vi "Initialize.vi"(8 "error in (no error)":errorcluster, 11 "Thread User Interface in":refnum<class "Thread User Interface.lvclass">) -> (0 "error out":errorcluster, 3 "Thread User Interface out":refnum<class "Thread User Interface.lvclass">)   [LabVIEW 2020, in "GE Reflective Memory.lvlib" / "Thread User Interface.lvclass"]
uses:
  Thread User Interface.lvclass
  Configurations/Thread/Thread Configuration.lvclass
  DSF Core.lvlibp/Classes/User Interface/User Interface.lvclass
  C:/Users/nitest/Desktop/Git 2020/niveristand-data-sharing-framework-custom-device-plugins/Components/DSF Core.lvlibp/Classes/Configuration/Configuration.lvclass
  C:/Users/nitest/Desktop/Git 2020/niveristand-data-sharing-framework-custom-device-plugins/Components/DSF Core.lvlibp/Classes/User Interface/User Interface.lvclass
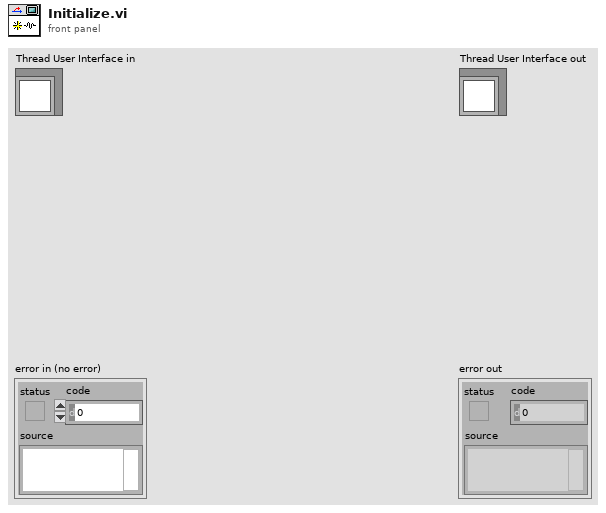
[diagram p1: front panel]
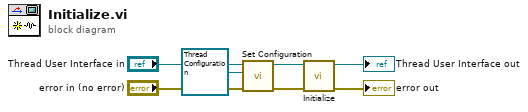
[diagram p0: block diagram]
diagram:
  n1 = call "Set Configuration.vi"("error in (no error)"="error in (no error)", "configuration"=refnum<class "Thread Configuration.lvclass"> refnum ("GE Reflective Memory.lvlib:Thread Configuration.lvclass"), "User Interface in"="Thread User Interface in") -> ("error out"=w3:errorcluster, "User Interface out"=w2:refnum<class "Thread User Interface.lvclass">)  [unwired: 7 in]
  n2 = call-parent "Initialize.vi"("error in (no error)"=w3, "User Interface in"=w2) -> ("error out"=→"error out":errorcluster, "User Interface out"=→"Thread User Interface out":refnum<class "Thread User Interface.lvclass">)  [unwired: 8 in]
